vi "Configure Channel (Off) Pulse.vi"(8 "error in (no error)":errorcluster, 10 "Channel (0001)":string="0001", 11 "VISA resource name":refnum<visa-resource-name>) -> (0 "error out":errorcluster, 2 "Channel":string, 3 "VISA resource name out":refnum<visa-resource-name>)   [LabVIEW 2020, in "Yokogawa GX Series.lvlib"]
doc: "Sets the input range as off (skip).\n\nCommand: SRangePulse"
uses:
  <instrlib>/Yokogawa GX Series/Yokogawa GX Series.lvlib
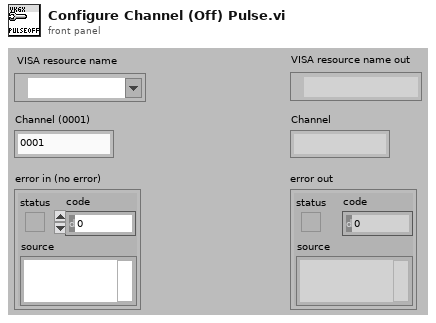
[diagram p1: front panel]
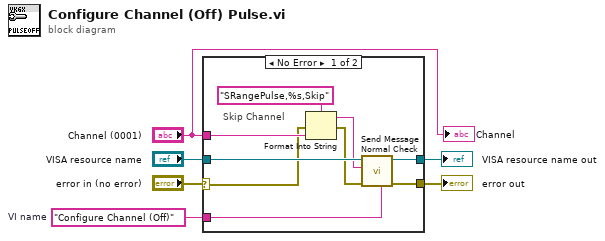
[diagram p0: block diagram]
diagram:
  w5 = "Configure Channel (Off)"  # VI name
  n1 = case shown="No Error" "error in (no error)" {
    selector: "error in (no error)" -> [w7 w16]
    tunnel: "VISA resource name" -> [w14 w17]
    tunnel: w5 -> [w12 _]
    tunnel: [w10 w17] -> w4
    tunnel: [w9 w16] -> w3
    tunnel: "Channel (0001)" -> [w8 _]
    frame No Error {
      # "Skip Channel"
      n2 = Format Into String(format string="SRangePulse,%s,Skip", error in=w7, w8) -> (resulting string=w11:string, error out=w13:errorcluster)  [unwired: 1 in]
      n3 = call <instrlib>:"Send Message Normal Check.vi"("Source (\"\")"=w12, "error in (no error)"=w13, "Send Message (\"\")"=w11, "VISA resource name"=w14) -> ("error out"=w9:errorcluster, "VISA resource name out"=w10:refnum<visa-resource-name>)  [unwired: 1 in, 5 out]
    }
    frame Error {
    }
  }
  "error out" <- w3
  "VISA resource name out" <- w4
  "Channel" <- "Channel (0001)"
